vi "ECS-1402-FPGA-EPTx.vi"() -> ()   [LabVIEW 2015, in "ECS-FPGA.lvlib"]
uses:
  ECS-FPGA.lvlib
  <vilib>/Powertrain Controls/Device Drivers/Engine Position Tracking/EPTx/RevA/FPGA/Controls/EPTxSupervisor.ctl
  <vilib>/Powertrain Controls/Device Drivers/Engine Position Tracking/EPTx/RevA/FPGA/Controls/EPTxConfig.ctl
  <vilib>/Powertrain Controls/Device Drivers/Engine Position Tracking/EPTx/RevA/FPGA/Controls/EPTxControl.ctl
  <vilib>/Powertrain Controls/Device Drivers/Engine Position Tracking/EPTx/RevA/FPGA/Controls/EPTxTooth.ctl
  <vilib>/Powertrain Controls/Device Drivers/Engine Position Tracking/EPTx/RevA/FPGA/Controls/EPTxAAPControl.ctl
  <vilib>/Powertrain Controls/Device Drivers/Engine Position Tracking/EPTx/RevA/FPGA/Controls/EPTxFuelSparkControl.ctl
  <vilib>/Platform/TimedLoop/XDataNode/timing_clust.ctl
  <vilib>/Platform/TimedLoop/XDataNode/nitl_modes.ctl
  <vilib>/Platform/TimedLoop/XDataNode/wakeup.ctl
  <vilib>/Powertrain Controls/Device Drivers/Engine Position Tracking/EPTx/RevA/FPGA/Controls/EPTxSignals.ctl
  <vilib>/rvi/Emulation/niFpgaSctlEmulationGetInTimedLoop.vi
  <vilib>/rvi/Emulation/niFpgaEmulationReportErrorSimple.vi
  <vilib>/rvi/Emulation/niFpgaGetClockAttributes.vi
  <vilib>/rvi/Emulation/niFpgaCriticalErrorInLSC.vi
  <vilib>/rvi/eio/common/nirviEmuTemplateMethod_errors.vi
  <vilib>/Platform/TimedLoop/XDataNode/XDataNode.xnode
  <vilib>/eio/EIONode/EIONode.xnode
  <vilib>/Platform/TimedLoop/XDataNode/XDNodeRunTimeDep.lvlib
  <vilib>/Powertrain Controls/Device Drivers/Engine Position Tracking/EPTx/RevA/FPGA/EPTx - RevA - FPGA.lvlib
panel:
  in  "O2-1.Control":T1
  out "O2-1.Data":T2
  in  "DI-1.PlsGen_Config_Channel3":T3
  in  "DI-1.PlsGen_Config_Channel2":T3
  in  "DI-1.PlsGen_Config_Channel1":T3
  in  "ESTTL-1.Sequences":T4(array[cluster])
  in  "ESTTL-1.Config":T5
  in  "PFI-1.FuelControl 4":T6
  in  "PFI-1.FuelControl 3":T6
  in  "PFI-1.FuelControl 2":T6
  in  "PFI-1.FuelControl 1":T6
  out "EPTx.Aux4CaptureCAD":fxp<+,18,11>
  out "EPTx.Aux3CaptureCAD":fxp<+,18,11>
  out "EPTx.Aux2CaptureCAD":fxp<+,18,11>
  out "EPTx.Aux1CaptureCAD":fxp<+,18,11>
  out "EPTx.Aux4EdgeCount":u8
  out "EPTx.Aux3EdgeCount":u8
  out "EPTx.Aux2EdgeCount":u8
  out "EPTx.Aux1EdgeCount":u8
  in  "EPTx.Aux4AngleCapture":T7
  in  "EPTx.Aux3AngleCapture":T7
  in  "EPTx.Aux2AngleCapture":T7
  in  "EPTx.Aux1AngleCapture":T7
  out "EPTxTooth":T8
  in  "EPTxControl":T9
  in  "EPTxConfig":T10
  out "EPTxSupervisor":T11
  out "ADCombo-1.DigitalTriggers":u32
  out "Throttle-1.Data":T12 caption="ThrottleData"
  in  "Throttle-1.Control":T13 caption="ThrottleControl"
  out "ADCombo-1.VRHallData":T14 caption="VRHallData"
  in  "EPTx.Aux4":u8=2
  in  "EPTx.Aux2":u8=1
  out "DI-1.Data":T15 caption="DIData"
  in  "ADCombo-1.VRHallInvert":u8
  in  "ADCombo-1.VR1.Filt":u16
  in  "ADCombo-1.VR2.Filt":u16
  in  "ADCombo-1.Hall1.Filt":u16
  in  "ADCombo-1.Hall2.Filt":u16
  in  "9411-1.0.Filt":u16
  in  "9411-1.1.Filt":u16
  in  "9411-1.2.Filt":u16
  in  "9411-1.3.Filt":u16
  in  "9411-1.4.Filt":u16
  in  "9411-1.5.Filt":u16
  in  "9411-1.Invert":u8
  out "ADCombo-1.ModulePresent":bool caption="ModulePresent"
  out "PFI-1.Data":T16 caption="PFIData"
  in  "PFI-1.IPhaseInterface":T17(array[cluster])=[{"IPhaseCurrent"=0, "IPhaseDuration"=0}, {"IPhaseCurrent"=0, "IPhaseDuration"=0}, {"IPhaseCurrent"=0, "IPhaseDuration"=0}, {"IPhaseCurrent"=0, "IPhaseDuration"=0}, {"IPhaseCurrent"=0, "IPhaseDuration"=0}, {"IPhaseCurrent"=0, "IPhaseDuration"=0}, {"IPhaseCurrent"=0, "IPhaseDuration"=0}, {"IPhaseCurrent"=0, "IPhaseDuration"=0}] caption="IPhaseInterface"
  in  "PFI-1.LowsidePWM":T18 caption="LowsidePWM"
  in  "PFI-1.Control":T19 caption="PFIControl"
  out "DI-1.ScopeData":T20 caption="DIScopeData"
  in  "DI-1.ScopeRead":bool caption="DIScopeRead"
  in  "DI-1.IPhaseInterface":T21(array[cluster]) caption="IPhaseInterface"
  in  "DI-1.Control":T22 caption="DIControl"
  in  "EPTx.Aux3":u8
  in  "EPTx.Primary":u8
  in  "EPTx.Aux1":u8
  out "ADCombo-1.Hall1.PPWData":T23
  out "ADCombo-1.Hall2.PPWData":T23
  out "ADCombo-1.VR2.PPWData":T23
  out "ADCombo-1.VR1.PPWData":T23
  out "9411-1.0.PPWData":T23
  out "9411-1.1.PPWData":T23
  out "9411-1.2.PPWData":T23
  out "9411-1.3.PPWData":T23
  out "9411-1.4.PPWData":T23
  out "9411-1.5.PPWData":T23
  out "9411-1.DigitalTriggers":u32
  out "ADCombo-1.AnalogData":T24 caption="AnalogData"
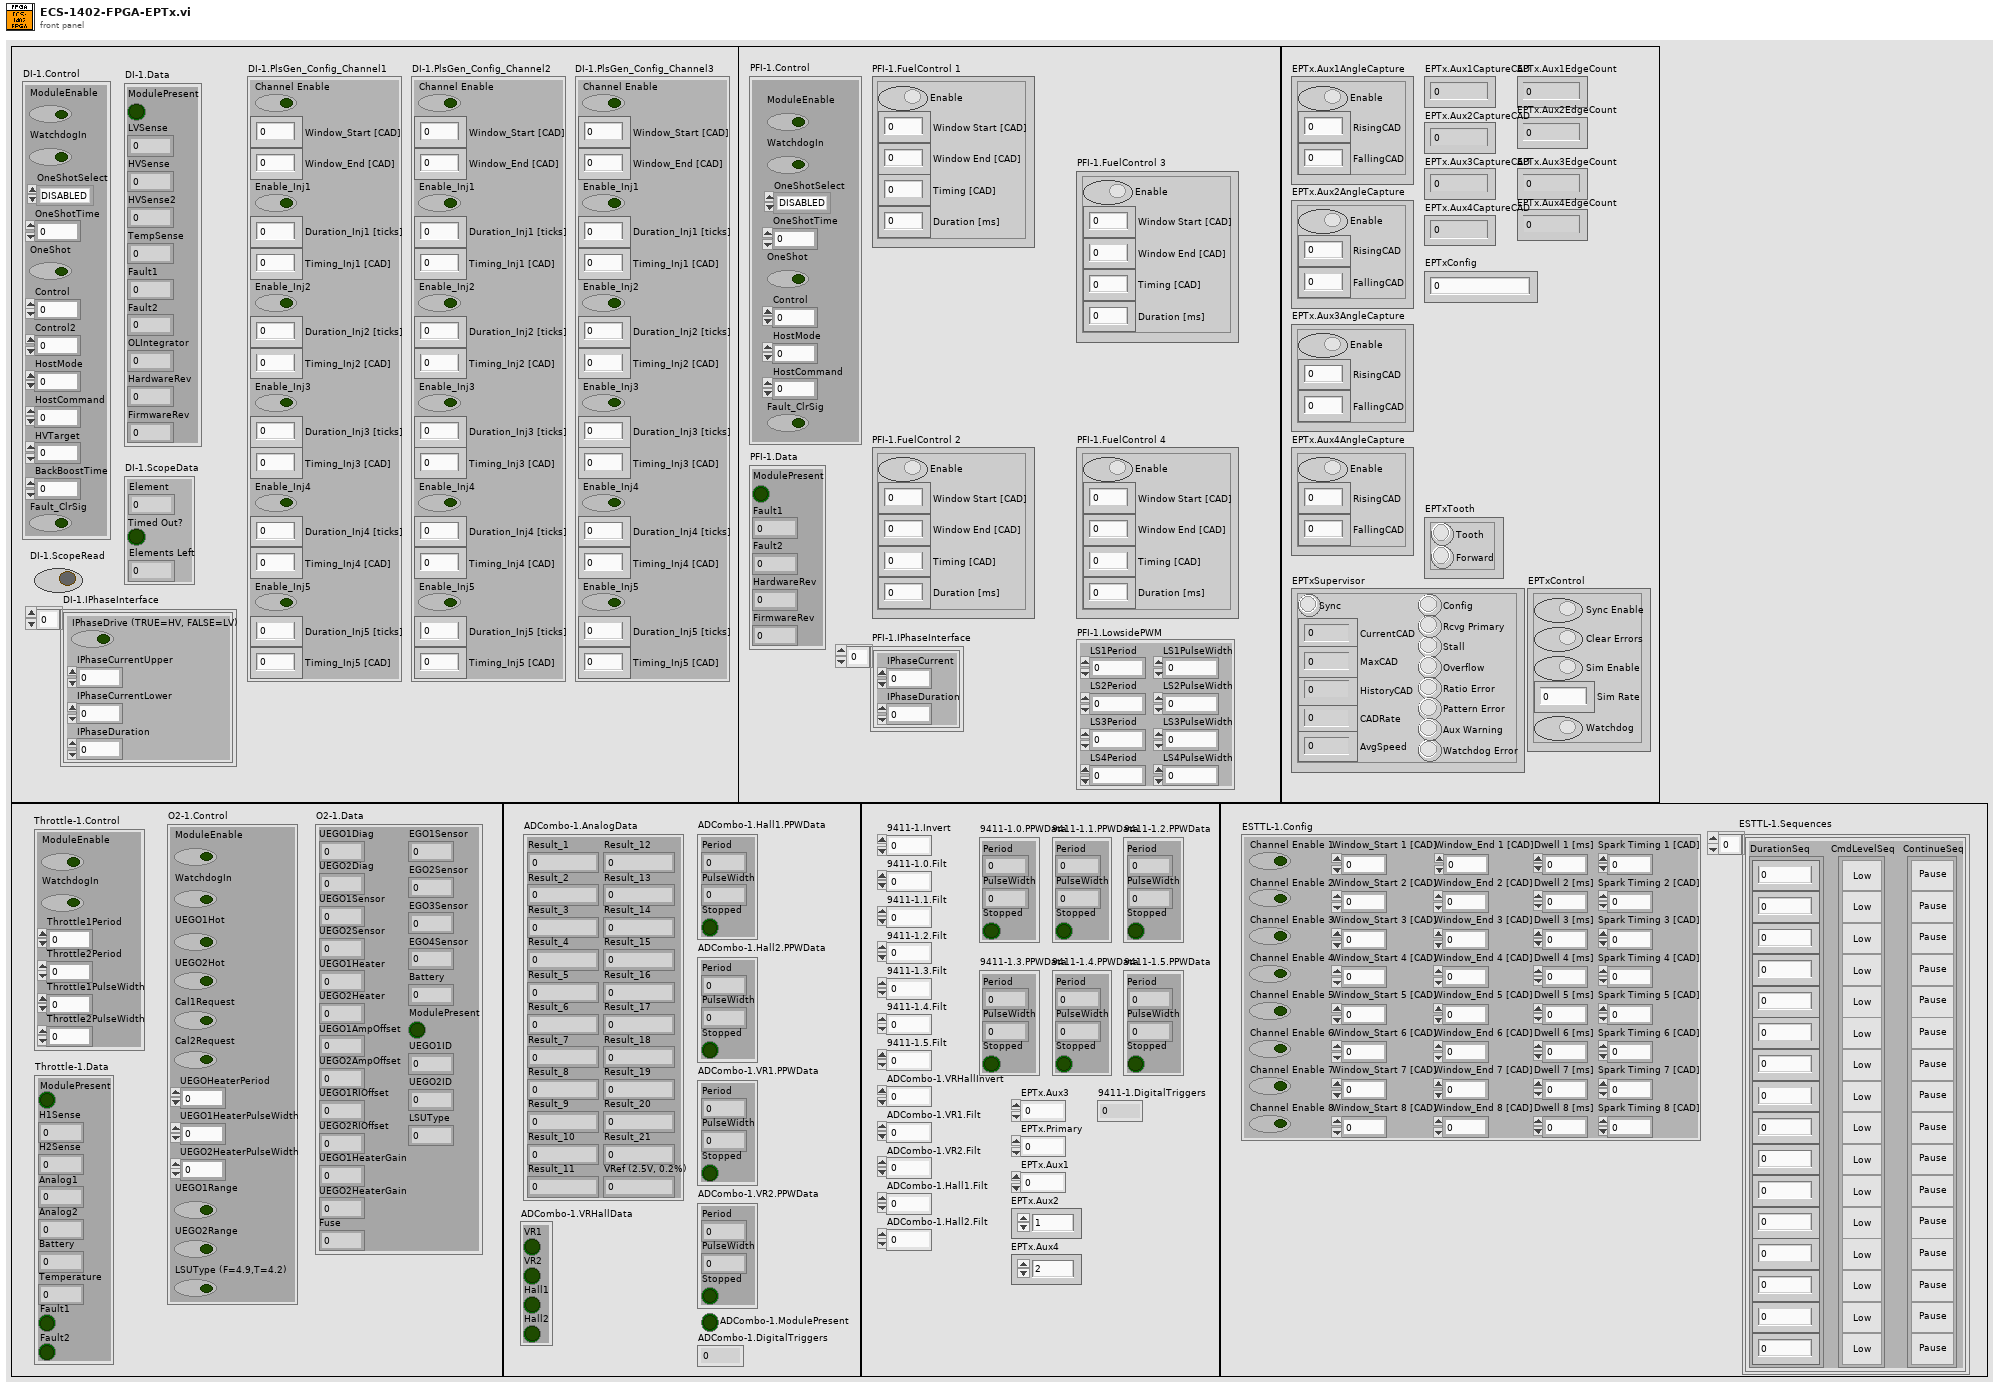
[diagram p1: front panel]
types:
  T1 = cluster{"ModuleEnable":bool, "WatchdogIn":bool, "UEGO1Hot":bool, "UEGO2Hot":bool, "Cal1Request":bool, "Cal2Request":bool, "UEGOHeaterPeriod":u16, "UEGO1HeaterPulseWidth":u16, "UEGO2HeaterPulseWidth":u16, "UEGO1Range":bool, "UEGO2Range":bool, "LSUType (F=4.9,T=4.2)":bool}
  T2 = cluster{"UEGO1Diag":u8, "UEGO2Diag":u8, "UEGO1Sensor":u16, "UEGO2Sensor":u16, "UEGO1Heater":u16, "UEGO2Heater":u16, "UEGO1AmpOffset":u16, "UEGO2AmpOffset":u16, "UEGO1RIOffset":u16, "UEGO2RIOffset":u16, "UEGO1HeaterGain":u16, "UEGO2HeaterGain":u16, "Fuse":u16, "EGO1Sensor":u16, "EGO2Sensor":u16, "EGO3Sensor":u16, "EGO4Sensor":u16, "Battery":u16, "ModulePresent":bool, "UEGO1ID":u8, "UEGO2ID":u8, "LSUType":u8}
  T3 = cluster{"Channel Enable":bool, "Window_Start [CAD]":fxp<+,18,11>, "Window_End [CAD]":fxp<+,18,11>, "Enable_Inj1":bool, "Duration_Inj1 [ticks]":u32, "Timing_Inj1 [CAD]":fxp<+,18,11>, "Enable_Inj2":bool, "Duration_Inj2 [ticks]":u32, "Timing_Inj2 [CAD]":fxp<+,18,11>, "Enable_Inj3":bool, "Duration_Inj3 [ticks]":u32, "Timing_Inj3 [CAD]":fxp<+,18,11>, "Enable_Inj4":bool, "Duration_Inj4 [ticks]":u32, "Timing_Inj4 [CAD]":fxp<+,18,11>, "Enable_Inj5":bool, "Duration_Inj5 [ticks]":u32, "Timing_Inj5 [CAD]":fxp<+,18,11>}
  T4 = cluster{"DurationSeq":u32[], "CmdLevelSeq":bool[], "ContinueSeq":bool[]}[]
  T5 = cluster{"Channel Enable 1":bool, "Window_Start 1 [CAD]":fxp<+,18,11>, "Window_End 1 [CAD]":fxp<+,18,11>, "Dwell 1 [ms]":fxp<+/-,22,9>, "Spark Timing 1 [CAD]":fxp<+,18,11>, "Channel Enable 2":bool, "Window_Start 2 [CAD]":fxp<+,18,11>, "Window_End 2 [CAD]":fxp<+,18,11>, "Dwell 2 [ms]":fxp<+/-,22,9>, "Spark Timing 2 [CAD]":fxp<+,18,11>, "Channel Enable 3":bool, "Window_Start 3 [CAD]":fxp<+,18,11>, "Window_End 3 [CAD]":fxp<+,18,11>, "Dwell 3 [ms]":fxp<+/-,22,9>, "Spark Timing 3 [CAD]":fxp<+,18,11>, "Channel Enable 4":bool, "Window_Start 4 [CAD]":fxp<+,18,11>, "Window_End 4 [CAD]":fxp<+,18,11>, "Dwell 4 [ms]":fxp<+/-,22,9>, "Spark Timing 4 [CAD]":fxp<+,18,11>, "Channel Enable 5":bool, "Window_Start 5 [CAD]":fxp<+,18,11>, "Window_End 5 [CAD]":fxp<+,18,11>, "Dwell 5 [ms]":fxp<+/-,22,9>, "Spark Timing 5 [CAD]":fxp<+,18,11>, "Channel Enable 6":bool, "Window_Start 6 [CAD]":fxp<+,18,11>, "Window_End 6 [CAD]":fxp<+,18,11>, "Dwell 6 [ms]":fxp<+/-,22,9>, "Spark Timing 6 [CAD]":fxp<+,18,11>, "Channel Enable 7":bool, "Window_Start 7 [CAD]":fxp<+,18,11>, "Window_End 7 [CAD]":fxp<+,18,11>, "Dwell 7 [ms]":fxp<+/-,22,9>, "Spark Timing 7 [CAD]":fxp<+,18,11>, "Channel Enable 8":bool, "Window_Start 8 [CAD]":fxp<+,18,11>, "Window_End 8 [CAD]":fxp<+,18,11>, "Dwell 8 [ms]":fxp<+/-,22,9>, "Spark Timing 8 [CAD]":fxp<+,18,11>}
  T6 = typedef "EPTx - RevA - FPGA.lvlib/EPTxFuelSparkControl.ctl" = cluster{"Enable":bool, "Window Start [CAD]":fxp<+,18,11>, "Window End [CAD]":fxp<+,18,11>, "Timing [CAD]":fxp<+,18,11>, "Duration [ms]":fxp<+/-,22,9>}
  T7 = typedef "EPTx - RevA - FPGA.lvlib/EPTxAAPControl.ctl" = cluster{"Enable":bool, "RisingCAD":fxp<+,18,11>, "FallingCAD":fxp<+,18,11>}
  T8 = typedef "EPTx - RevA - FPGA.lvlib/EPTxTooth.ctl" = cluster{"Tooth":bool, "Forward":bool}
  T9 = typedef "EPTx - RevA - FPGA.lvlib/EPTxControl.ctl" = cluster{"Sync Enable":bool, "Clear Errors":bool, "Sim Enable":bool, "Sim Rate":fxp<+,24,6>, "Watchdog":bool}
  T10 = typedef "EPTx - RevA - FPGA.lvlib/EPTxConfig.ctl" = u64
  T11 = typedef "EPTx - RevA - FPGA.lvlib/EPTxSupervisor.ctl" = cluster{"Sync":bool, "CurrentCAD":fxp<+,18,11>, "MaxCAD":fxp<+,11,11>, "HistoryCAD":fxp<+,11,11>, "CADRate":fxp<+,22,8>, "AvgSpeed":fxp<+,17,15>, "Config":bool, "Rcvg Primary":bool, "Stall":bool, "Overflow":bool, "Ratio Error":bool, "Pattern Error":bool, "Aux Warning":bool, "Watchdog Error":bool}
  T12 = cluster{"ModulePresent":bool, "H1Sense":i16, "H2Sense":i16, "Analog1":i16, "Analog2":i16, "Battery":i16, "Temperature":i16, "Fault1":bool, "Fault2":bool}
  T13 = cluster{"ModuleEnable":bool, "WatchdogIn":bool, "Throttle1Period":u16, "Throttle2Period":u16, "Throttle1PulseWidth":i16, "Throttle2PulseWidth":i16}
  T14 = cluster{"VR1":bool, "VR2":bool, "Hall1":bool, "Hall2":bool}
  T15 = cluster{"ModulePresent":bool, "LVSense":u8, "HVSense":u8, "HVSense2":u8, "TempSense":i8, "Fault1":u8, "Fault2":u8, "OLIntegrator":u32, "HardwareRev":u8, "FirmwareRev":u8}
  T16 = cluster{"ModulePresent":bool, "Fault1":u8, "Fault2":u8, "HardwareRev":u8, "FirmwareRev":u8}
  T17 = cluster{"IPhaseCurrent":u16, "IPhaseDuration":u16}[]
  T18 = cluster{"LS1Period":u32, "LS1PulseWidth":u32, "LS2Period":u32, "LS2PulseWidth":u32, "LS3Period":u32, "LS3PulseWidth":u32, "LS4Period":u32, "LS4PulseWidth":u32}
  T19 = cluster{"ModuleEnable":bool, "WatchdogIn":bool, "OneShotSelect":enum8{"DISABLED", "PFI 1", "PFI 2", "PFI 3", "PFI 4"}, "OneShotTime":u32, "OneShot":bool, "Control":u16, "HostMode":u8, "HostCommand":u32, "Fault_ClrSig":bool}
  T20 = cluster{"Element":u32, "Timed Out?":bool, "Elements Left":u32}
  T21 = cluster{"IPhaseDrive (TRUE=HV, FALSE=LV)":bool, "IPhaseCurrentUpper":u16, "IPhaseCurrentLower":u16, "IPhaseDuration":u16}[]
  T22 = cluster{"ModuleEnable":bool, "WatchdogIn":bool, "OneShotSelect":enum8{"DISABLED", "CHAN 1", "CHAN 2", "CHAN 3"}, "OneShotTime":u32, "OneShot":bool, "Control":u8, "Control2":u8, "HostMode":u8, "HostCommand":u32, "HVTarget":u8, "BackBoostTime":u8, "Fault_ClrSig":bool}
  T23 = cluster{"Period":u32, "PulseWidth":u32, "Stopped":bool}
  T24 = cluster{"Result_1":u16, "Result_2":u16, "Result_3":u16, "Result_4":u16, "Result_5":u16, "Result_6":u16, "Result_7":u16, "Result_8":u16, "Result_9":u16, "Result_10":u16, "Result_11":u16, "Result_12":u16, "Result_13":u16, "Result_14":u16, "Result_15":u16, "Result_16":u16, "Result_17":u16, "Result_18":u16, "Result_19":u16, "Result_20":u16, "Result_21":u16, "VRef (2.5V, 0.2%)":u16}
  T25 = typedef "XDNodeRunTimeDep.lvlib/timing_clust.ctl" = cluster{"Expected End [f-1]":u64, "Actual End [f-1]":u64, "Finished Late? [f-1]":bool, "Expected End [i-1]":u64, "Actual End [i-1]":u64, "Finished Late? [i-1]":bool, "Expected Start [i]":u64, "Actual Start [i]":u64, "Expected Start [f]":u64, "Actual Start [f]":u64, "Source Name":string, "Structure Name":string, "Period":i64, "Deadline":i64, "Offset":i64, "Start":i64, "Priority":i32, "Timeout":i32, "Mode":T26, "Wakeup Reason":T27, "Error":errorcluster, "Source Type":string, "Secondary Source Type":string, "Global End Time":u64, "Global Start Time":u64, "Frame Duration":u64, "Iteration Duration":u64, "Assigned CPU":i32, "I/O Scan Engine Mode":u32}
  T26 = typedef "XDNodeRunTimeDep.lvlib/nitl_modes.ctl" = enum32{"No Change", "Process missed periods, maintain original phase", "Discard missed periods, maintain original phase", "Process missed periods, ignore original phase", "Discard missed periods, ignore original phase"}
  T27 = typedef "XDNodeRunTimeDep.lvlib/wakeup.ctl" = enum32{"Normal", "Aborted", "Asynchronous wakeup", "Timing source error", "Timed loop error", "Timeout"}
  T28 = typedef "EPTx - RevA - FPGA.lvlib/EPTxSignals.ctl" = cluster{"Primary":bool, "Aux 1":bool, "Aux 2":bool, "Aux 3":bool, "Aux 4":bool}
  T29 = cluster{"CmdOut1":bool, "CmdOut2":bool, "CmdOut3":bool, "CmdOut4":bool, "CmdOut5":bool, "CmdOut6":bool, "CmdOut7":bool, "CmdOut8":bool}
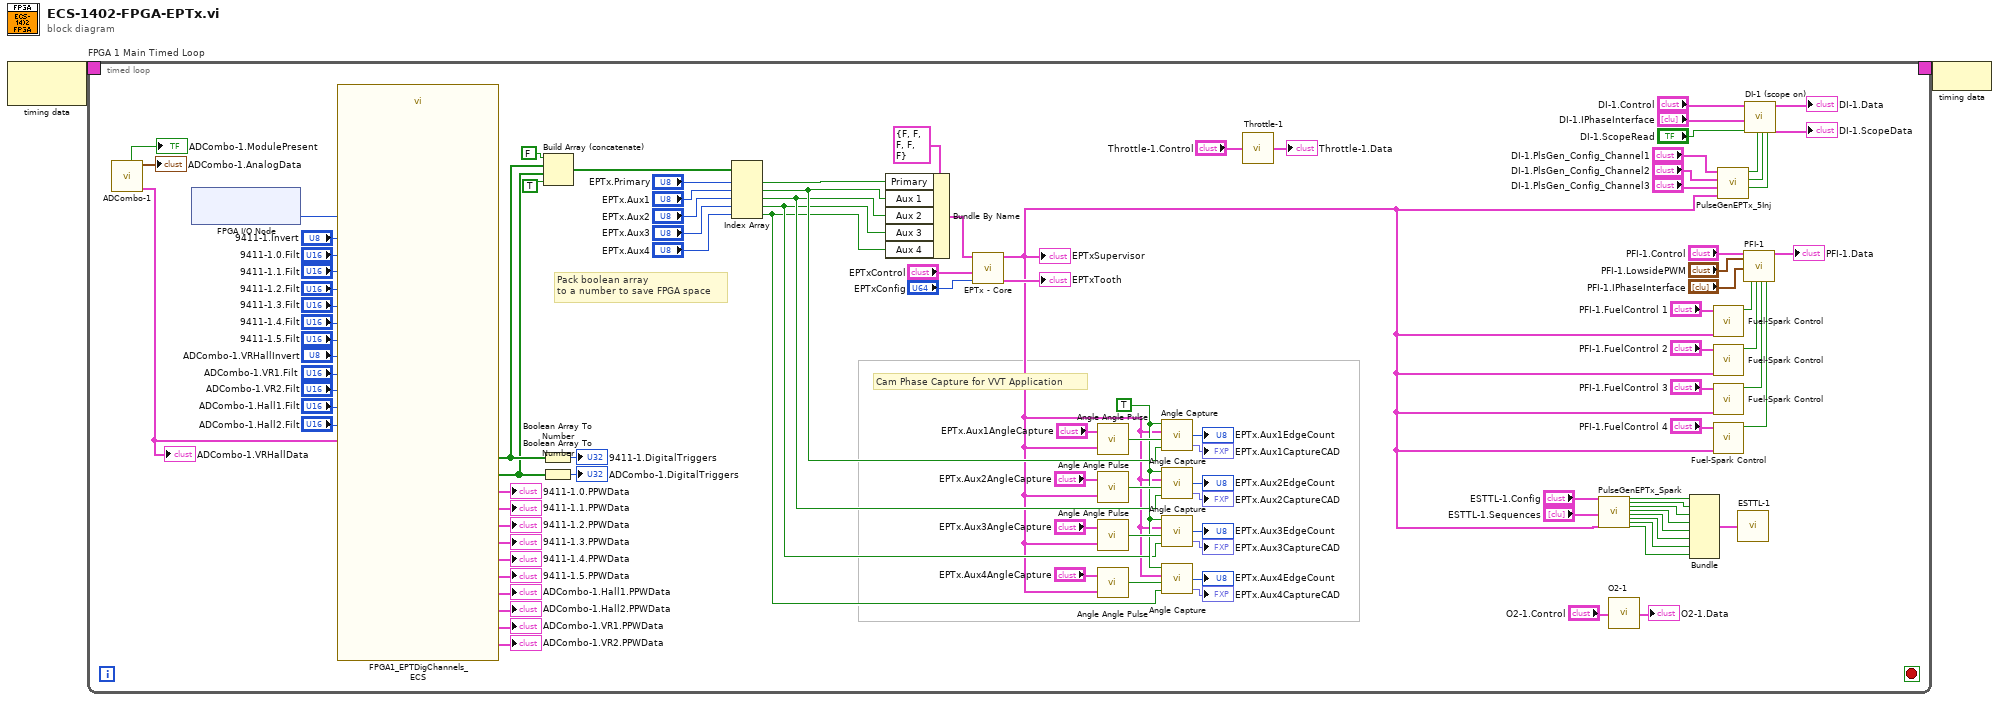
[diagram p0: block diagram]
diagram:
  n1 = node-c288() -> (w2:T25)  [unwired: 1 in]
  n2 = timed-loop "FPGA 1 Main Timed Loop" {
    timing: w2 -> [_]
    timing-out: [_] -> w1
    stop <- _ stop-if-true
    w44 = TRUE ("Enable")
    # "Pack boolean array\nto a number to save FPGA space"
    # "Cam Phase Capture for VVT Application"
    n3 = call "ADCombo-1"() -> ("ADCombo-1_VRHallData"=w106:T14, "ADCombo-1_AnalogData"=→"ADCombo-1.AnalogData":T24, "ADCombo-1_ModulePresent"=→"ADCombo-1.ModulePresent":bool)  [unwired: 5 in, 2 out]
    "ADCombo-1.VRHallData" <- w106
    n4 = xnode "FPGA I/O Node"() -> ("9411-1/DI5:0"=w103:u8)  [unwired: 1 in, 1 out]
    n5 = call "FPGA1_EPTDigChannels_ECS.vi"("NI9411-1.2.Filt"="9411-1.2.Filt", "NI9411-1.3.Filt"="9411-1.3.Filt", "NI9411-1.4.Filt"="9411-1.4.Filt", "NI9411-1.5.Filt"="9411-1.5.Filt", "ADCombo-1.VRHallData"=w106, "ADCombo-1.VR1.Filt"="ADCombo-1.VR1.Filt", "ADCombo-1.VR2.Filt"="ADCombo-1.VR2.Filt", "9411/DI5:0"=w103, "ADCombo-1.Hall1.Filt"="ADCombo-1.Hall1.Filt", "NI9411-1.1.Filt"="9411-1.1.Filt", "ADCombo-1.Hall2.Filt"="ADCombo-1.Hall2.Filt", "NI9411-1.Invert"="9411-1.Invert", "ADCombo-1.VRHallInvert"="ADCombo-1.VRHallInvert", "NI9411-1.0.Filt"="9411-1.0.Filt") -> ("9411-1.0.PPWData"=→"9411-1.0.PPWData":T23, "ADCombo-1.Hall2.PPWData"=→"ADCombo-1.Hall2.PPWData":T23, "9411-1.1.PPWData"=→"9411-1.1.PPWData":T23, "ADCombo-1.Hall1.PPWData"=→"ADCombo-1.Hall1.PPWData":T23, "9411-1.2.PPWData"=→"9411-1.2.PPWData":T23, "9411-1.3.PPWData"=→"9411-1.3.PPWData":T23, "9411-1.4.PPWData"=→"9411-1.4.PPWData":T23, "9411-1.5.PPWData"=→"9411-1.5.PPWData":T23, "9411-1.DigitalTriggers"=w62:bool[], "ADCombo-1.VR1.PPWData"=→"ADCombo-1.VR1.PPWData":T23, "ADCombo-1.VR2.PPWData"=→"ADCombo-1.VR2.PPWData":T23, "ADCombo-1.DigitalTriggers"=w61:bool[])  [unwired: 2 in]
    n6 = Boolean Array To Number(Boolean array=w62) -> (number=→"9411-1.DigitalTriggers":u32)
    n7 = Boolean Array To Number(Boolean array=w61) -> (number=→"ADCombo-1.DigitalTriggers":u32)
    n8 = Build Array (concatenate)(FALSE, w62, w61, TRUE) -> (w53:bool[])
    n9 = Index Array(array=w53, index #1="EPTx.Primary", index #2="EPTx.Aux1", index #3="EPTx.Aux2", index #4="EPTx.Aux3", index #5="EPTx.Aux4") -> (element #1=w24:bool, element #2=w23:bool, element #3=w22:bool, element #4=w21:bool, element #5=w20:bool)
    n10 = Bundle By Name(cluster=T28 {"Primary"=FALSE, "Aux 1"=FALSE, "Aux 2"=FALSE, "Aux 3"=FALSE, "Aux 4"=FALSE} ("EPTxSignals"), "Primary"=w24, "Aux 1"=w23, "Aux 2"=w22, "Aux 3"=w21, "Aux 4"=w20) -> (w55:T28)
    n11 = call <vilib>:"EPTx - Core.vi"("EPTxConfig"="EPTxConfig", "EPTxControl"="EPTxControl", "EPTxSignals"=w55) -> ("EPTxTooth"=→"EPTxTooth":T8, "EPTxSupervisor"=w8:T11)  [unwired: 7 in]
    "EPTxSupervisor" <- w8
    n12 = call <vilib>:"Angle Angle Pulse.vi"("EPTxSupervisor"=w8, "AAPControl"="EPTx.Aux1AngleCapture") -> ("AAP"=w50:bool)
    n13 = call <vilib>:"Angle Angle Pulse.vi"("EPTxSupervisor"=w8, "AAPControl"="EPTx.Aux2AngleCapture") -> ("AAP"=w49:bool)
    n14 = call <vilib>:"Angle Angle Pulse.vi"("EPTxSupervisor"=w8, "AAPControl"="EPTx.Aux3AngleCapture") -> ("AAP"=w48:bool)
    n15 = call <vilib>:"Angle Angle Pulse.vi"("EPTxSupervisor"=w8, "AAPControl"="EPTx.Aux4AngleCapture") -> ("AAP"=w45:bool)
    n16 = call <vilib>:"Angle Capture.vi"("Capture"=w23, "OpWindow"=w50, "EPTxSupervisor"=w8, "Enable"=w44) -> ("CaptureCAD"=→"EPTx.Aux1CaptureCAD":fxp<+,18,11>, "CaptureCount"=→"EPTx.Aux1EdgeCount":u8)  [unwired: 1 out]
    n17 = call <vilib>:"Angle Capture.vi"("Capture"=w22, "OpWindow"=w49, "EPTxSupervisor"=w8, "Enable"=w44) -> ("CaptureCAD"=→"EPTx.Aux2CaptureCAD":fxp<+,18,11>, "CaptureCount"=→"EPTx.Aux2EdgeCount":u8)  [unwired: 1 out]
    n18 = call <vilib>:"Angle Capture.vi"("Capture"=w21, "OpWindow"=w48, "EPTxSupervisor"=w8, "Enable"=w44) -> ("CaptureCAD"=→"EPTx.Aux3CaptureCAD":fxp<+,18,11>, "CaptureCount"=→"EPTx.Aux3EdgeCount":u8)  [unwired: 1 out]
    n19 = call <vilib>:"Angle Capture.vi"("Capture"=w20, "OpWindow"=w45, "EPTxSupervisor"=w8, "Enable"=w44) -> ("CaptureCAD"=→"EPTx.Aux4CaptureCAD":fxp<+,18,11>, "CaptureCount"=→"EPTx.Aux4EdgeCount":u8)  [unwired: 1 out]
    n20 = call "Throttle-1"("Throttle-1_Control"="Throttle-1.Control") -> ("Throttle-1_Data"=→"Throttle-1.Data":T12)
    n21 = call "PulseGenEPTx_Spark.vi"("Spark_Config"="ESTTL-1.Config", "Spark_Sequences"="ESTTL-1.Sequences", "EPTxSupervisor"=w8) -> ("CmdOut1"=w19:bool, "CmdOut2"=w18:bool, "CmdOut3"=w17:bool, "CmdOut4"=w16:bool, "CmdOut5"=w15:bool, "CmdOut6"=w14:bool, "CmdOut7"=w13:bool, "CmdOut8"=w12:bool)  [unwired: 17 in]
    n22 = call "O2-1"("O2Control"="O2-1.Control") -> ("O2Data"=→"O2-1.Data":T2)
    n23 = Bundle("CmdOut1"=w19, "CmdOut2"=w18, "CmdOut3"=w17, "CmdOut4"=w16, "CmdOut5"=w15, "CmdOut6"=w14, "CmdOut7"=w13, "CmdOut8"=w12) -> (w11:T29)  [unwired: 1 out]
    n24 = call <vilib>:"Fuel-Spark Control.vi"("EPTxSupervisor"=w8, "Fuel-Spark Control"="PFI-1.FuelControl 1") -> ("Fuel-Spark Command"=w25:bool)  [unwired: 9 in]
    n25 = call <vilib>:"Fuel-Spark Control.vi"("EPTxSupervisor"=w8, "Fuel-Spark Control"="PFI-1.FuelControl 2") -> ("Fuel-Spark Command"=w26:bool)  [unwired: 9 in]
    n26 = call <vilib>:"Fuel-Spark Control.vi"("EPTxSupervisor"=w8, "Fuel-Spark Control"="PFI-1.FuelControl 3") -> ("Fuel-Spark Command"=w27:bool)  [unwired: 9 in]
    n27 = call <vilib>:"Fuel-Spark Control.vi"("EPTxSupervisor"=w8, "Fuel-Spark Control"="PFI-1.FuelControl 4") -> ("Fuel-Spark Command"=w28:bool)  [unwired: 9 in]
    n28 = call "PulseGenEPTx_5Inj.vi"("EPTxSupervisor"=w8, "Inj_Config_Channel3"="DI-1.PlsGen_Config_Channel3", "Inj_Config_Channel2"="DI-1.PlsGen_Config_Channel2", "Inj_Config_Channel1"="DI-1.PlsGen_Config_Channel1") -> ("CmdOut3"=w33:bool, "CmdOut2"=w34:bool, "CmdOut1"=w35:bool)  [unwired: 3 in]
    n29 = call "ESTTL-1"("ESTTL-1_ESTTLChan"=w11) -> ()  [unwired: 1 out]
    n30 = call "PFI-1"("PFI-1_Control"="PFI-1.Control", "PFI-1_LowsidePWM"="PFI-1.LowsidePWM", "PFI-1_IPhaseInterface"="PFI-1.IPhaseInterface", "PFI1Cmd"=w25, "PFI2Cmd"=w26, "PFI3Cmd"=w27, "PFI4Cmd"=w28) -> ("PFI-1_Data"=→"PFI-1.Data":T16)  [unwired: 11 in, 1 out]
    n31 = call "DI-1 (scope on)"("DI-1_Control"="DI-1.Control", "DI-1_IPhaseInterface"="DI-1.IPhaseInterface", "DI-1_ScopeRead"="DI-1.ScopeRead", "DI1Cmd"=w35, "DI2Cmd"=w34, "DI3Cmd"=w33) -> ("DI-1_Data"=→"DI-1.Data":T15, "DI-1_ScopeData"=→"DI-1.ScopeData":T20)  [unwired: 11 in, 1 out]
  }
  n32 = node-c288(w1) -> ()
